vi "TOF cal new.vi"() -> ()   [LabVIEW 2014]
uses:
  <vilib>/Analysis/NI_AALPro.lvlib
panel:
  out "TOF OF DHB 2":dbl
  in  "Table Control":string[][](table)
  out "TOF OF POTASSIUM":dbl
  out "TOF OF SODIUM":dbl
  out "TOF OF DHB DIMER":dbl
  out "TOF OF THE FRAGMENT":dbl
  in  "CHARGE OF THE FRAGMENT":dbl
  in  "MASS OF FRAGMENT":dbl
  out "TOF OF DEH. DHB":dbl
  out "TOF OF DHB":dbl
  out "TOF OF INDIUM":dbl
  out "TOF OF TETRA CATION FROM OFFSET":dbl
  out "TOF OF TRICATION FROM OFFSET":dbl
  out "TOF OF DICATION FROM OFFSET":dbl
  out "TOF OF MOLECULE FROM OFFSET":dbl
  in  "MASS OF FRAGMENT  O4":dbl
  in  "MASS OF FRAGMENT  O3":dbl
  in  "MASS  OF FRAGMENT  O2":dbl
  in  "MASS  OF FRAGMENT O1":dbl
  in  "tof of fragment O4":dbl
  in  "tof of fragment O3":dbl
  in  "tof of fragment O2":dbl
  in  "tof of fragment O1":dbl
  out "TOF OF Cu":dbl
  out "TOF OF IRON":dbl
  out "MASS  OF FRAGMENT  4":dbl
  out "MASS OF FRAGMENT  3":dbl
  out "MASS  OF FRAGMENT  2":dbl
  out "MASS OF FRAGMENT -1":dbl
  in  "tof of fragment 4":dbl
  in  "tof of fragment 3":dbl
  in  "tof of fragment 2":dbl
  in  "tof of fragment 1":dbl
  out "TOF OF TETRA CATION":dbl
  out "TOF OF TRICATION":dbl
  out "TOF OF DICATION":dbl
  out "TOF OF MOLECULE":dbl
  in  "TOF of known fragment":dbl
  in  "mass of known fragment":dbl
  in  "?":u16(ring) items=["Hydrogen", "Helium", "Argon", "Krypton", "Xenon", "1,3-butadiene", "Water", "Methyl Iodide", "Ethane"]
  in  "?":bool
  # "TIME OF FLIGHT CALCULATOR"
  # "SELECT THE REFERENCE"
  # "TOF OF COMMON MOLECULES"
  # "SELECT THE MOLECULE"
  # "TOF OF SINGLE CATION"
  # "TOF OF IRON"
  # "TOF OF DHB (154)"
  # "TOF OF CHC (154)"
  # "ENTER MASS OF CUSTOM FRAGMENT"
  # "TOF OF DICATION"
  # "TOF OF COPPER"
  # "TOF OF DEH. DHB (137)"
  # "ENTER TOF OF THE REFERNCE"
  # "TOF OF TRI CATION"
  # "TOF OF INDIUM (114.8)"
  # "TOF OF DHB DIMER (237)"
  # "TOF OF TETRA CATION"
  # "TOF OF SOIDUM (23)"
  # "TOF OF POTASSIUM (39)"
  # "OFFSET CALCULATOR"
  # "TOF OF CALCULATOR"
  # "MASS CALCULATOR"
  # "ENTER TOF OF \nFRAGMENT - 1"
  # "ENTER TOF OF \nFRAGMENT - 1"
  # "MASS OF FRAGMENT - 1"
  # "MASS OF FRAGMENT - 1"
  # "TOF OF SINGLE CATION"
  # "ENTER TOF OF \nFRAGMENT - 2"
  # "ENTER TOF OF \nFRAGMENT - 2"
  # "MASS OF FRAGMENT - 2"
  # "MASS OF FRAGMENT - 2"
  # "TOF OF DICATION"
  # "ENTER TOF OF \nFRAGMENT - 3"
  # "ENTER TOF OF \nFRAGMENT - 3"
  # "MASS OF FRAGMENT - 3"
  # "MASS OF FRAGMENT - 3"
  # "TOF OF TRI CATION"
  # "ENTER TOF OF \nFRAGMENT - 4"
  # "ENTER TOF OF \nFRAGMENT - 4"
  # "MASS OF FRAGMENT - 4"
  # "MASS OF FRAGMENT - 4"
  # "TOF OF TETRA CATION"
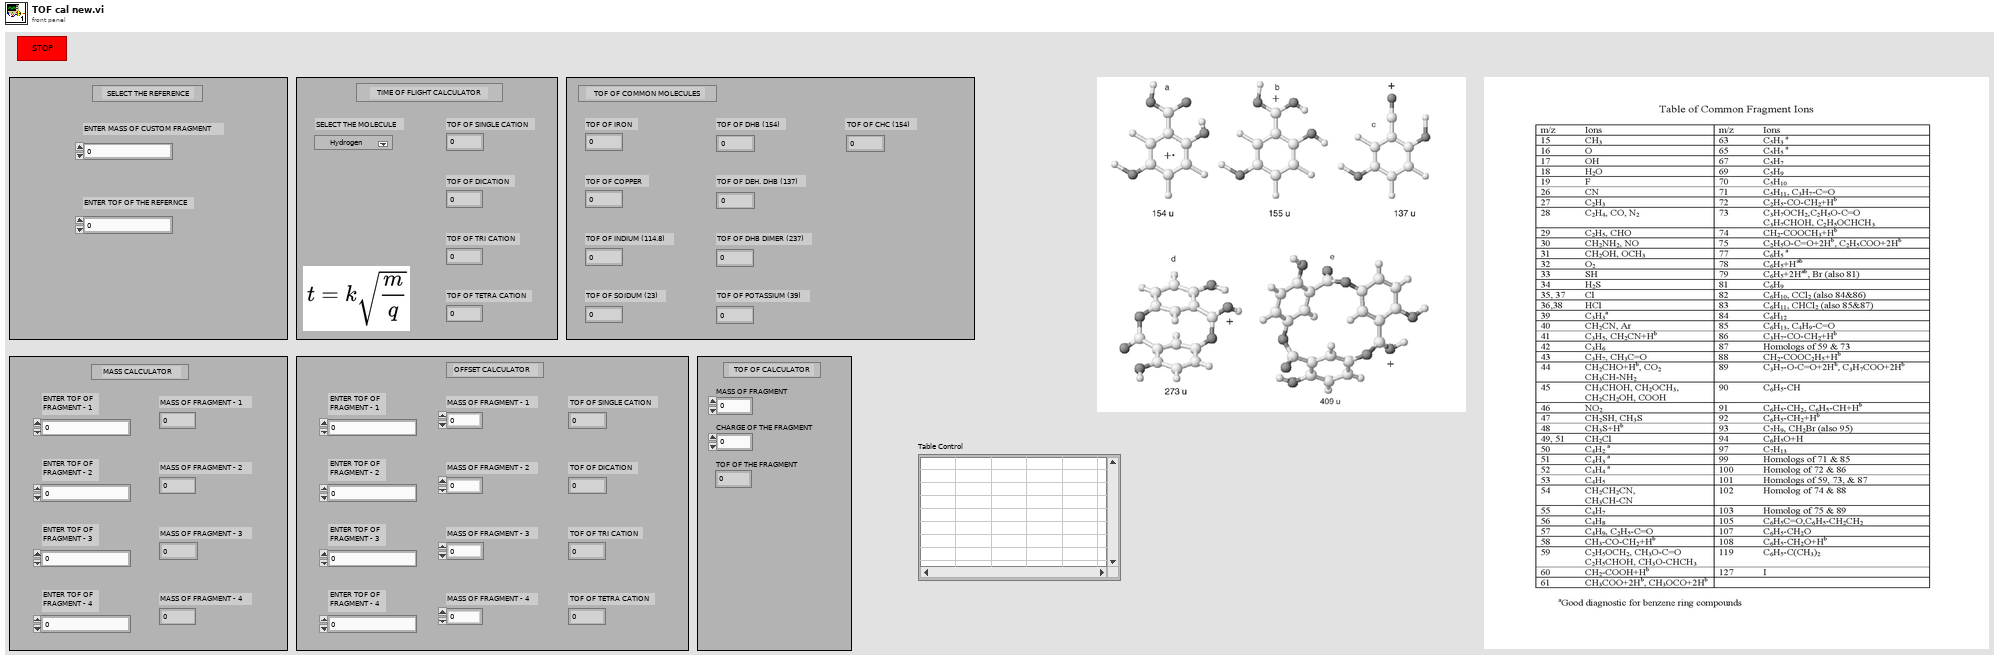
[diagram p1: front panel]
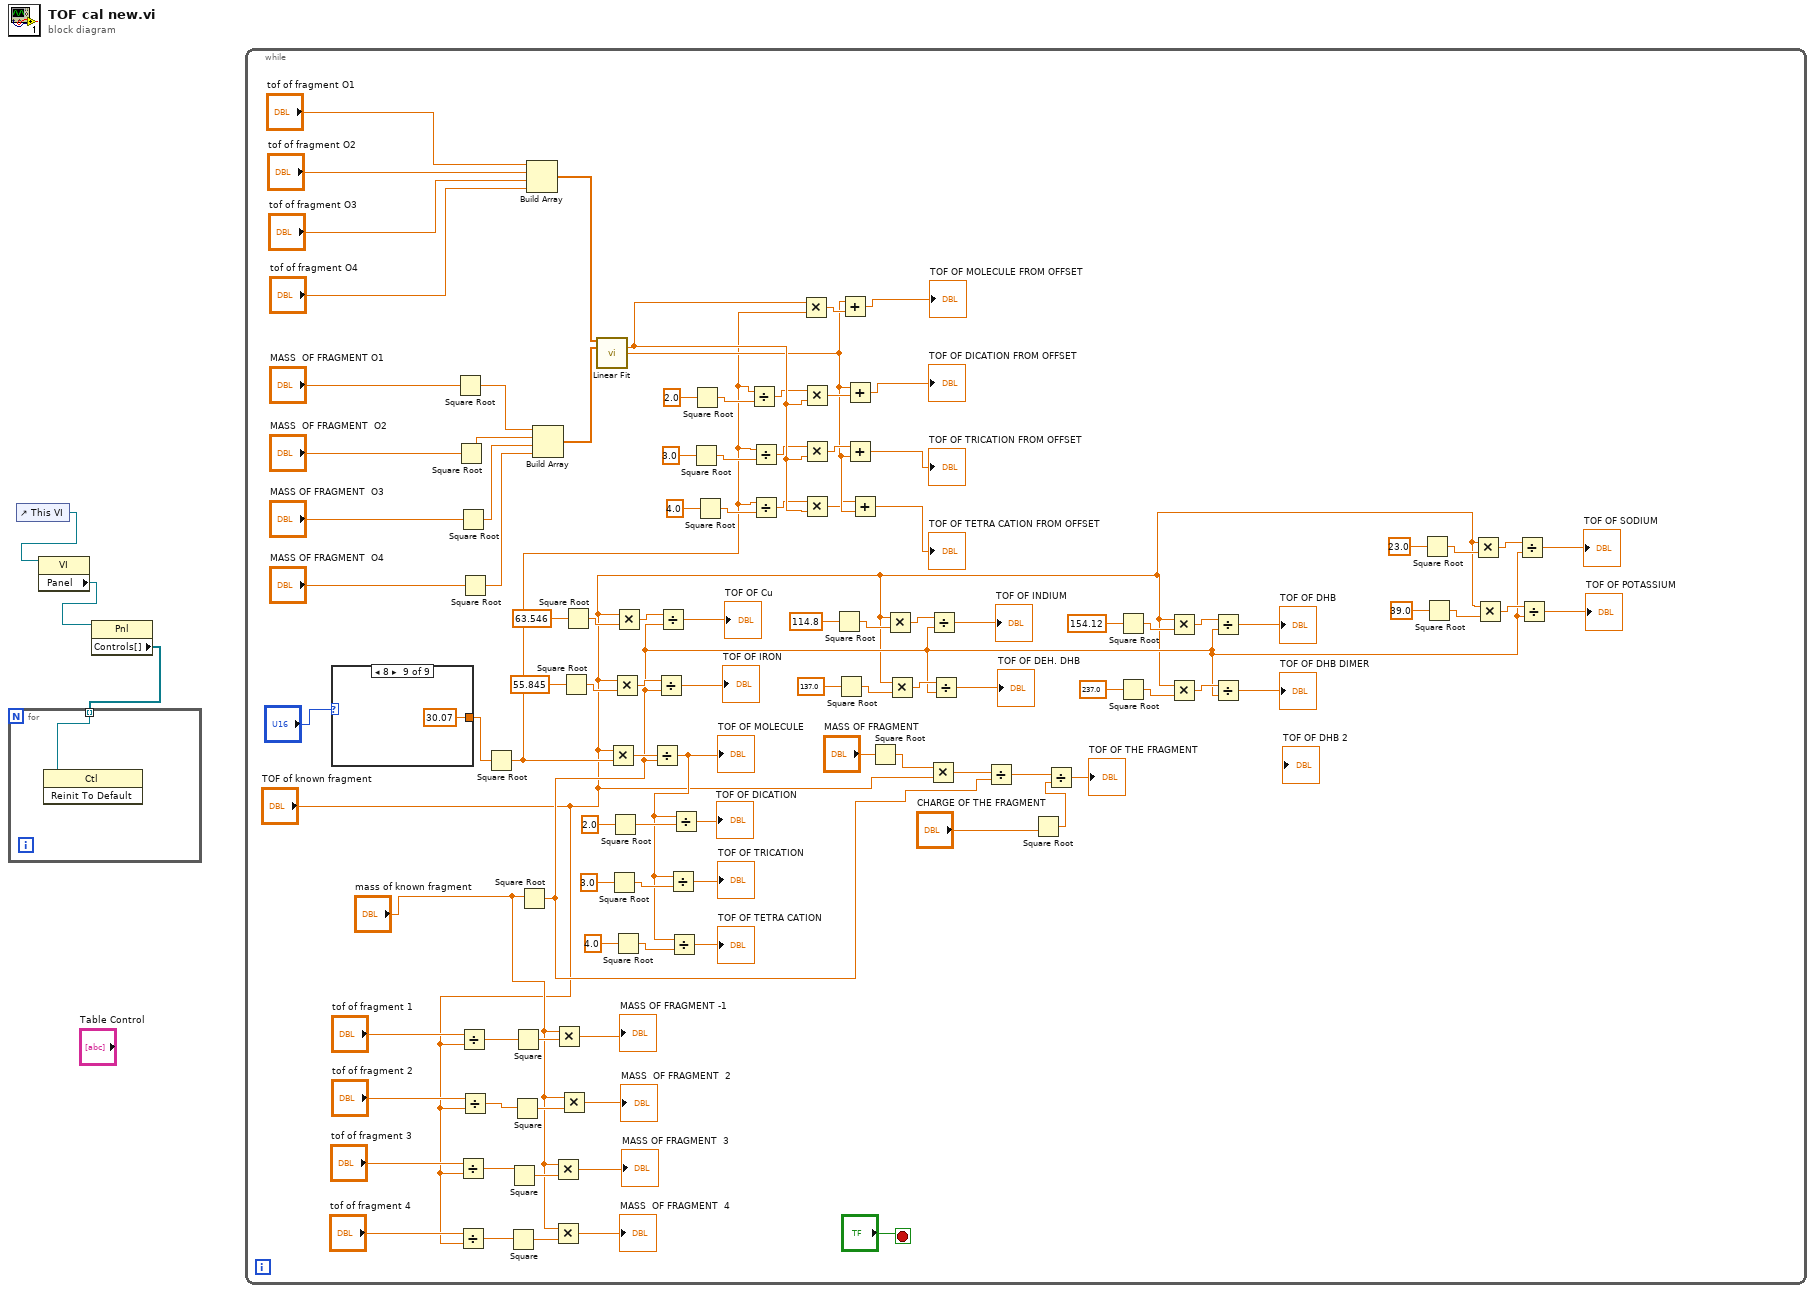
[diagram p0: block diagram]
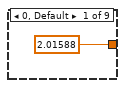
[diagram p2: hidden frame]
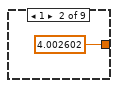
[diagram p3: hidden frame]
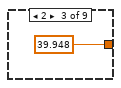
[diagram p4: hidden frame]
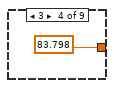
[diagram p5: hidden frame]
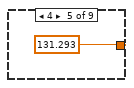
[diagram p6: hidden frame]
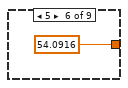
[diagram p7: hidden frame]
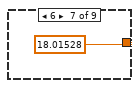
[diagram p8: hidden frame]
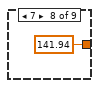
[diagram p9: hidden frame]
diagram:
  n1 = control-ref of="This VI"() -> (w3:refnum<vi>)
  n2 = property class="VI"(reference=w3) -> ("Panel"=w2:refnum<vi>)  [unwired: 1 in, 2 out]
  n3 = property class="Pnl"(reference=w2) -> ("Controls[]"=w1:refnum<vi>[])  [unwired: 1 in, 2 out]
  n4 = for {
    tunnel: w1 -> [w4] mode=indexing
    n5 = invoke class="Ctl" method="Reinit To Default"(reference=w4) -> ()  [unwired: 2 in, 3 out]
  }
  n6 = while {
    stop <- "?" stop-if-true
    n7 = case shown="8" "?" {
      tunnel: [2.01588 4.002602 39.948 83.798 131.293 54.0916 18.01528 ("Enter the Molar Mass \nof Frgament/Molecule/Element") 141.94 ("Enter the Molar Mass \nof Frgament/Molecule/Element") 30.07 ("Enter the Molar Mass \nof Frgament/Molecule/Element")] -> w58
      frame 0, Default {
      }
      frame 1 {
      }
      frame 2 {
      }
      frame 3 {
      }
      frame 4 {
      }
      frame 5 {
      }
      frame 6 {
      }
      frame 7 {
      }
      frame 8 {
      }
    }
    n8 = Square Root(x="MASS  OF FRAGMENT O1") -> (sqrt(x)=w68:dbl)
    n9 = Square Root(x="MASS  OF FRAGMENT  O2") -> (sqrt(x)=w67:dbl)
    n10 = Square Root(x="MASS OF FRAGMENT  O3") -> (sqrt(x)=w66:dbl)
    n11 = Divide(x="tof of fragment 3", y="TOF of known fragment") -> (x/y=w91:dbl)
    n12 = Divide(x="tof of fragment 4", y="TOF of known fragment") -> (x/y=w90:dbl)
    n13 = Divide(x="tof of fragment 1", y="TOF of known fragment") -> (x/y=w93:dbl)
    n14 = Square Root(x="MASS OF FRAGMENT  O4") -> (sqrt(x)=w65:dbl)
    n15 = Divide(x="tof of fragment 2", y="TOF of known fragment") -> (x/y=w92:dbl)
    n16 = Square Root(x=w58) -> (sqrt(x)=w36:dbl)
    n17 = Square(x=w90) -> (x^2=w85:dbl)
    n18 = Square(x=w91) -> (x^2=w88:dbl)
    n19 = Square(x=w92) -> (x^2=w87:dbl)
    n20 = Square(x=w93) -> (x^2=w89:dbl)
    n21 = Square Root(x="mass of known fragment") -> (sqrt(x)=w6:dbl)
    n22 = Build Array("tof of fragment O1", "tof of fragment O2", "tof of fragment O3", "tof of fragment O4") -> (w60:dbl[])
    n23 = Build Array(w68, w67, w66, w65) -> (w59:dbl[])
    n24 = Multiply(x="mass of known fragment", y=w88) -> (x*y=→"MASS OF FRAGMENT  3":dbl)
    n25 = Multiply(x="mass of known fragment", y=w85) -> (x*y=→"MASS  OF FRAGMENT  4":dbl)
    n26 = Multiply(x="mass of known fragment", y=w89) -> (x*y=→"MASS OF FRAGMENT -1":dbl)
    n27 = Multiply(x="mass of known fragment", y=w87) -> (x*y=→"MASS  OF FRAGMENT  2":dbl)
    n28 = Square Root(x=55.845) -> (sqrt(x)=w77:dbl)
    n29 = Square Root(x=63.546) -> (sqrt(x)=w78:dbl)
    n30 = call <vilib>:"Linear Fit.vi"("Y"=w60, "X"=w59) -> ("slope"=w51:dbl, "intercept"=w44:dbl)  [unwired: 9 in, 3 out]
    n31 = Multiply(x="TOF of known fragment", y=w36) -> (x*y=w108:dbl)
    n32 = Square Root(x=3.0) -> (sqrt(x)=w106:dbl)
    n33 = Square Root(x=2.0) -> (sqrt(x)=w107:dbl)
    n34 = Multiply(x="TOF of known fragment", y=w77) -> (x*y=w75:dbl)
    n35 = Square Root(x=4.0) -> (sqrt(x)=w105:dbl)
    n36 = Multiply(x="TOF of known fragment", y=w78) -> (x*y=w76:dbl)
    n37 = Divide(x=w108, y=w6) -> (x/y=w101:dbl)
    "TOF OF MOLECULE" <- w101
    n38 = Divide(x=w75, y=w6) -> (x/y=→"TOF OF IRON":dbl)
    n39 = Divide(x=w76, y=w6) -> (x/y=→"TOF OF Cu":dbl)
    n40 = Divide(x=w101, y=w106) -> (x/y=→"TOF OF TRICATION":dbl)
    n41 = Divide(x=w101, y=w105) -> (x/y=→"TOF OF TETRA CATION":dbl)
    n42 = Divide(x=w101, y=w107) -> (x/y=→"TOF OF DICATION":dbl)
    n43 = Square Root(x=3.0) -> (sqrt(x)=w53:dbl)
    n44 = Square Root(x=2.0) -> (sqrt(x)=w52:dbl)
    n45 = Square Root(x=4.0) -> (sqrt(x)=w54:dbl)
    n46 = Divide(x=w36, y=w52) -> (x/y=w50:dbl)
    n47 = Divide(x=w36, y=w53) -> (x/y=w49:dbl)
    n48 = Divide(x=w36, y=w54) -> (x/y=w48:dbl)
    n49 = Multiply(x=w51, y=w36) -> (x*y=w45:dbl)
    n50 = Multiply(x=w50, y=w51) -> (x*y=w46:dbl)
    n51 = Multiply(x=w49, y=w51) -> (x*y=w47:dbl)
    n52 = Multiply(x=w48, y=w51) -> (x*y=w43:dbl)
    n53 = Square Root(x=114.8) -> (sqrt(x)=w29:dbl)
    n54 = Square Root(x=137.0) -> (sqrt(x)=w25:dbl)
    n55 = Add(x=w44, y=w45) -> (x+y=→"TOF OF MOLECULE FROM OFFSET":dbl)
    n56 = Add(x=w44, y=w46) -> (x+y=→"TOF OF DICATION FROM OFFSET":dbl)
    n57 = Add(x=w47, y=w44) -> (x+y=→"TOF OF TRICATION FROM OFFSET":dbl)
    n58 = Add(x=w43, y=w44) -> (x+y=→"TOF OF TETRA CATION FROM OFFSET":dbl)
    n59 = Square Root(x="MASS OF FRAGMENT") -> (sqrt(x)=w38:dbl)
    n60 = Multiply(x="TOF of known fragment", y=w29) -> (x*y=w28:dbl)
    n61 = Multiply(x="TOF of known fragment", y=w25) -> (x*y=w24:dbl)
    n62 = Multiply(x=w38, y="TOF of known fragment") -> (x*y=w31:dbl)
    n63 = Divide(x=w28, y=w6) -> (x/y=→"TOF OF INDIUM":dbl)
    n64 = Divide(x=w24, y=w6) -> (x/y=→"TOF OF DEH. DHB":dbl)
    n65 = Divide(x=w31, y=w6) -> (x/y=w33:dbl)
    n66 = Square Root(x="CHARGE OF THE FRAGMENT") -> (sqrt(x)=w34:dbl)
    n67 = Divide(x=w33, y=w34) -> (x/y=→"TOF OF THE FRAGMENT":dbl)
    n68 = Square Root(x=154.12) -> (sqrt(x)=w21:dbl)
    n69 = Square Root(x=237.0) -> (sqrt(x)=w17:dbl)
    n70 = Multiply(x="TOF of known fragment", y=w21) -> (x*y=w20:dbl)
    n71 = Multiply(x="TOF of known fragment", y=w17) -> (x*y=w16:dbl)
    n72 = Divide(x=w20, y=w6) -> (x/y=→"TOF OF DHB":dbl)
    n73 = Divide(x=w16, y=w6) -> (x/y=→"TOF OF DHB DIMER":dbl)
    n74 = Square Root(x=23.0) -> (sqrt(x)=w13:dbl)
    n75 = Square Root(x=39.0) -> (sqrt(x)=w9:dbl)
    n76 = Multiply(x="TOF of known fragment", y=w13) -> (x*y=w12:dbl)
    n77 = Multiply(x="TOF of known fragment", y=w9) -> (x*y=w8:dbl)
    n78 = Divide(x=w12, y=w6) -> (x/y=→"TOF OF SODIUM":dbl)
    n79 = Divide(x=w8, y=w6) -> (x/y=→"TOF OF POTASSIUM":dbl)
  }
